vi "niFPGA 32-Bit Cast Specify Component.vi"(0 "Specify Component Info In":refnum<class "SpecComp(DiagramComp).lvclass">, 11 "error in (no error)":errorcluster) -> (4 "Specify Component Info Out":refnum<class "SpecComp(DiagramComp).lvclass">, 15 "error out":errorcluster)   [LabVIEW 2017]
uses:
  <vilib>/rvi/ClientSDK/Core/ModuleGeneration/ClassModGen/SpecifyComponent(DiagramComponent)/SpecComp(DiagramComp).lvclass
  e:/penguin/lvdist/win32/export/17.0/17.0.1f1/dist/vi.lib/rvi/ClientSDK/Core/ModuleGeneration/ClassModGen/SpecifyComponent/SpecifyComponent.lvclass
  <vilib>/rvi/ClientSDK/Core/ModuleGeneration/ClassModGen/SpecifyComponent/SpecifyComponent.lvclass
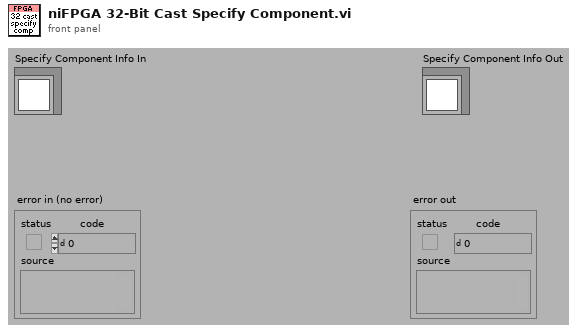
[diagram p1: front panel]
types:
  T1 = typedef "nirviModTimingInfo.ctl" = T2[]
  T2 = typedef "nirviModInfoPortTiming.ctl" = cluster{"Port Name":string, "Recall\nNeeded":bool, "Single Cycle Info":cluster{"Support Single Cycle Loops":bool, "Contains Embedded Shift Reg":bool, "Logic/Time Estimate":i32}, "Async Info":cluster{"Support Async Operation":bool, "Logic/Time Estimate":i32}, "Normal Info":cluster{"Support Normal Enable":bool, "Support Pulse Enable":bool, "Logic/Time Estimate":i32, "IO Offset":i32, "Pipeline Depth":i32, "Init Time Needed":i32}}
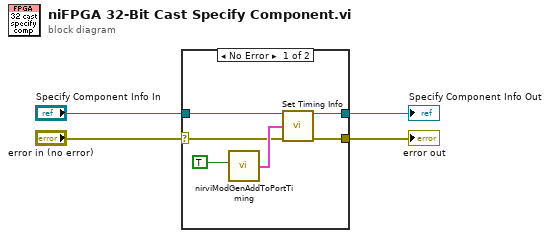
[diagram p0: block diagram]
diagram:
  n1 = case shown="No Error" "error in (no error)" {
    selector: "error in (no error)" -> [w8 w12]
    tunnel: [w5 w12] -> w3
    tunnel: "Specify Component Info In" -> [w7 w11]
    tunnel: [w6 w11] -> w1
    frame No Error {
      n2 = call <vilib>:"nirviModGenAddToPortTiming.vi"("Support Single Cycle Loops"=TRUE) -> ("Timing Info Out"=w10:T1)  [unwired: 5 in]
      n3 = call <vilib>:"Set Timing Info.vi"("ModGenInfo in"=w7, "Timing Info"=w10, "error in (no error)"=w8) -> ("ModGenInfo out"=w6:refnum<class "SpecComp(DiagramComp).lvclass">, "error out"=w5:errorcluster)  [unwired: 11 in]
    }
    frame Error {
    }
  }
  "error out" <- w3
  "Specify Component Info Out" <- w1
